vi "Read ColorString.vi"(8 "error in (no error)":errorcluster, 11 "Paint in":refnum<class "Paint.lvclass">) -> (0 "error out":errorcluster, 2 "ColorString":string, 3 "Paint out":refnum<class "Paint.lvclass">)   [LabVIEW 2014, in "Paint.lvclass"]
uses:
  Paint.lvclass
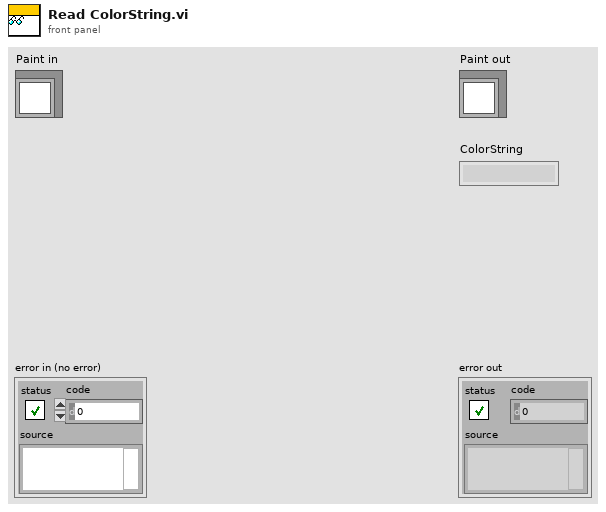
[diagram p1: front panel]
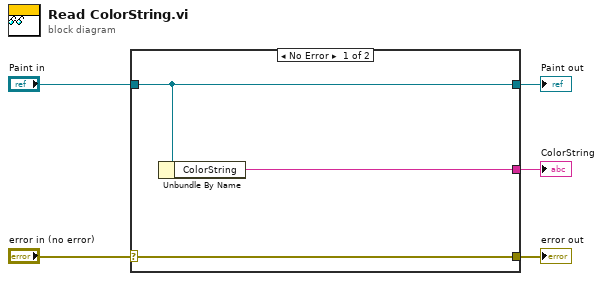
[diagram p0: block diagram]
diagram:
  n1 = case shown="No Error" "error in (no error)" {
    selector: "error in (no error)" -> [w8 w9]
    tunnel: [w8 w9] -> w4
    tunnel: [w7 w10] -> w2
    tunnel: "Paint in" -> [w7 w10]
    tunnel: [w6 _] -> w1
    frame No Error {
      n2 = Unbundle By Name(w7) -> ("ColorString"=w6:string)
    }
    frame Error {
    }
  }
  "error out" <- w4
  "Paint out" <- w2
  "ColorString" <- w1
